vi "init.vi"(8 "error in (no error)":errorcluster, 11 "Glaz-I in":refnum<class "Glaz.lvclass">) -> (0 "error out":errorcluster, 3 "Glaz-I out":refnum<class "Glaz.lvclass">)   [LabVIEW 2019, in "Glaz.lvclass"]
uses:
  Glaz.lvclass
  _cameraBase/_cameraBase.lvclass
panel:
  out "Hardware Version":string
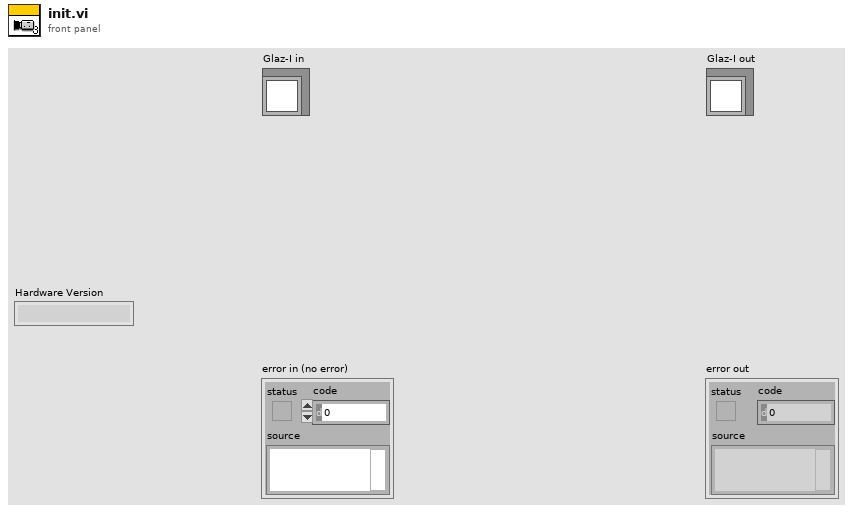
[diagram p1: front panel]
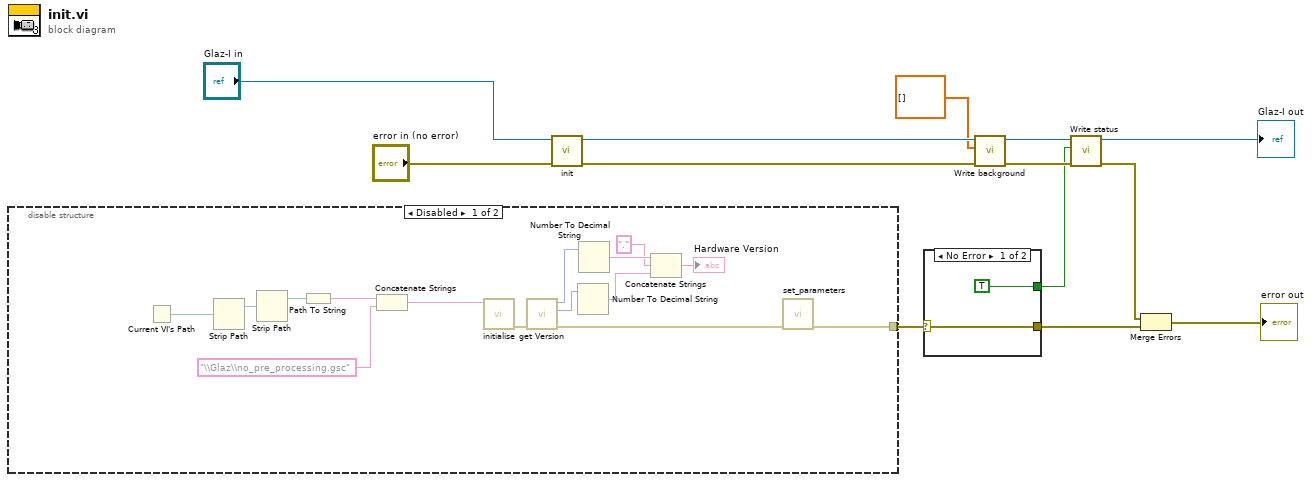
[diagram p0: block diagram]
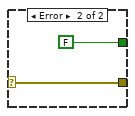
[diagram p3: hidden frame]
diagram:
  n1 = disable-structure shown="Disabled" {
    disable-tunnel: [w20 _] -> w7
    frame Disabled {
      n2 = Current VI's Path() -> (path=w19:path)
      n3 = Strip Path(path=w19) -> (stripped path=w18:path)  [unwired: 1 out]
      n4 = Strip Path(path=w18) -> (stripped path=w17:path)  [unwired: 1 out]
      n5 = Path To String(path=w17) -> (string=w16:string)
      n6 = Concatenate Strings(w16, "\\Glaz\\no_pre_processing.gsc") -> (w14:string)
      n7 = call <userlib>:"initialise.vi"("scriptFileName"=w14) -> ("error out"=w23:errorcluster)  [unwired: 9 in, 1 out]
      n8 = call <userlib>:"get Version.vi"("error in (no error)"=w23) -> ("error out"=w21:errorcluster, "minorVersion"=w25:i32, "majorVersion"=w24:i32)  [unwired: 8 in]
      n9 = Number To Decimal String(number=w25) -> (decimal integer string=w28:string)  [unwired: 1 in]
      n10 = Number To Decimal String(number=w24) -> (decimal integer string=w26:string)  [unwired: 1 in]
      n11 = Concatenate Strings(w26, "." ("string"), w28) -> (→"Hardware Version":string)
      n12 = call "set_parameters.vi"("error in (no error)"=w21) -> ("error out (no error)"=w20:errorcluster)  [unwired: 10 in]
    }
    frame Enabled {
    }
  }
  n13 = call-parent "init.vi"("error in (no error)"="error in (no error)", "_cameraBase in"="Glaz-I in") -> ("error out"=w9:errorcluster, "_cameraBase out"=w11:refnum<class "Glaz.lvclass">)  [unwired: 8 in]
  n14 = case shown="No Error" w7 {
    selector: w7 -> [w30 w32]
    tunnel: [w30 w32] -> w6
    tunnel: [TRUE FALSE] -> w1
    frame No Error {
    }
    frame Error {
    }
  }
  n15 = call-dynamic "Write background.vi"("error in (no error)"=w9, "background"=dbl[] [], "Glaz-I in"=w11) -> ("error out"=w4:errorcluster, "Glaz-I out"=w5:refnum<class "Glaz.lvclass">)  [unwired: 7 in]
  n16 = call-dynamic "Write status.vi"("error in (no error)"=w4, "status"=w1, "_cameraBase in"=w5) -> ("error out"=w2:errorcluster, "_cameraBase out"=→"Glaz-I out":refnum<class "Glaz.lvclass">)  [unwired: 7 in]
  n17 = Merge Errors(w2, w6) -> (→"error out":errorcluster)
